vi "Read configuration.vi"(8 "error in":errorcluster, 11 "LED editor node in":refnum<class "LED editor node.lvclass">) -> (0 "error out":errorcluster, 2 "configuration":refnum<class "NISE_CEF_serializable configuration.lvclass">, 3 "LED editor node out":refnum<class "LED editor node.lvclass">)   [LabVIEW 2014, in "LED editor node.lvclass"]
uses:
  LED editor node.lvclass
  <vilib>/NI/Configuration Framework/serializable configuration/NISE_CEF_serializable configuration.lvclass
  LED editor node.lvclass/LED editor node.ctl
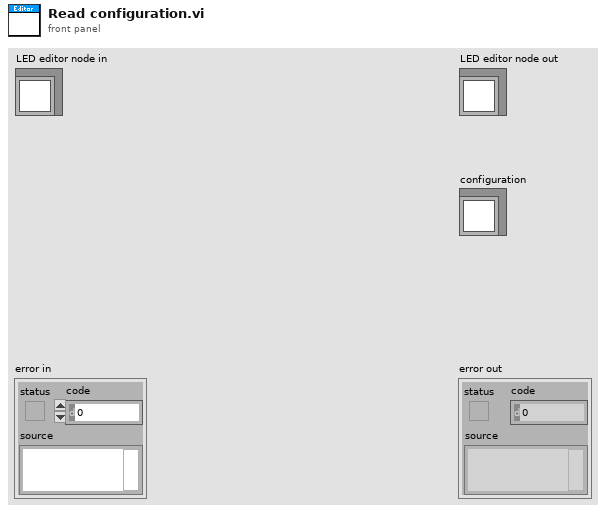
[diagram p1: front panel]
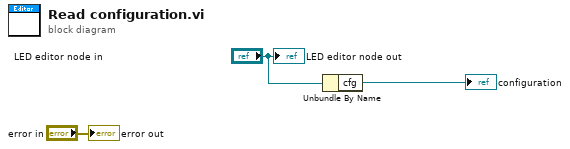
[diagram p0: block diagram]
diagram:
  n1 = Unbundle By Name("LED editor node in") -> ("cfg"=→"configuration":refnum<class "LED configuration.lvclass">)
  "error out" <- "error in"
  "LED editor node out" <- "LED editor node in"
